vi "PID control XY vel Z R.vi"(0 "x location (um)":dbl, 1 "x polarity":bool=TRUE, 2 "y polarity":bool, 3 "z polarity":bool, 5 "y location (um)":dbl, 7 "z location (um)":dbl, 9 "measurement time":dbl, 11 "reinitialize? (F)":bool, 12 "XY vel range (mm/s)":cluster{"output high":dbl, "output low":dbl}={"output high"=1000.0, "output low"=-1000.0} {"output low" format="%.2f"; "output high" format="%.2f"}, 13 "z position range (um)":cluster{"output high":dbl, "output low":dbl}={"output high"=100.0, "output low"=-100.0} {"output low" format="%.2f"; "output high" format="%.2f"}, 14 "XY gains":T2={"chase time (ms)"=200.0, "integral time (Ti, sec)"=1.0, "derivative time (Td, sec)"=0.0} {"derivative time (Td, sec)" format="%.3f"; "integral time (Ti, sec)" format="%.3f"; "chase time (ms)" format="%.3f"}, 15 "Z gains":T1={"proportional gain (Kc)"=0.7, "integral time (Ti, sec)"=1.0, "derivative time (Td, sec)"=0.0} {"derivative time (Td, sec)" format="%.3f"; "integral time (Ti, sec)" format="%.3f"; "proportional gain (Kc)" format="%.3f"}) -> (4 "x move (um)":dbl, 6 "y move (um)":dbl, 8 "z move (um)":dbl)   [LabVIEW 2010]
uses:
  <vilib>/addons/control/pid/pid.llb/PID (DBL Array).vi
  <vilib>/addons/control/pid/NI_PID_pid.lvlib
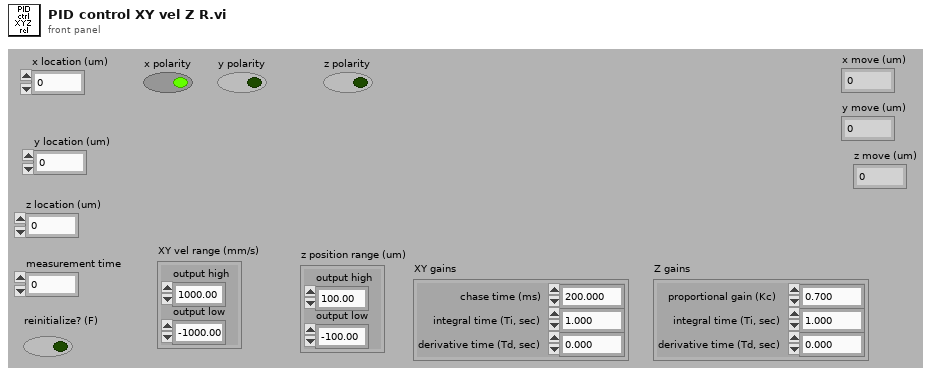
[diagram p1: front panel]
types:
  T1 = cluster{"proportional gain (Kc)":dbl, "integral time (Ti, sec)":dbl, "derivative time (Td, sec)":dbl}
  T2 = cluster{"chase time (ms)":dbl, "integral time (Ti, sec)":dbl, "derivative time (Td, sec)":dbl}
  T3 = cluster{"proportional gain (Kc)":dbl, "integral time (Ti, min)":dbl, "derivative time (Td, min)":dbl}
  T4 = cluster{"proportional gain (Kc)":dbl, "integral time (Ti, min)":dbl, "derivative time (Td, min)":dbl}[]
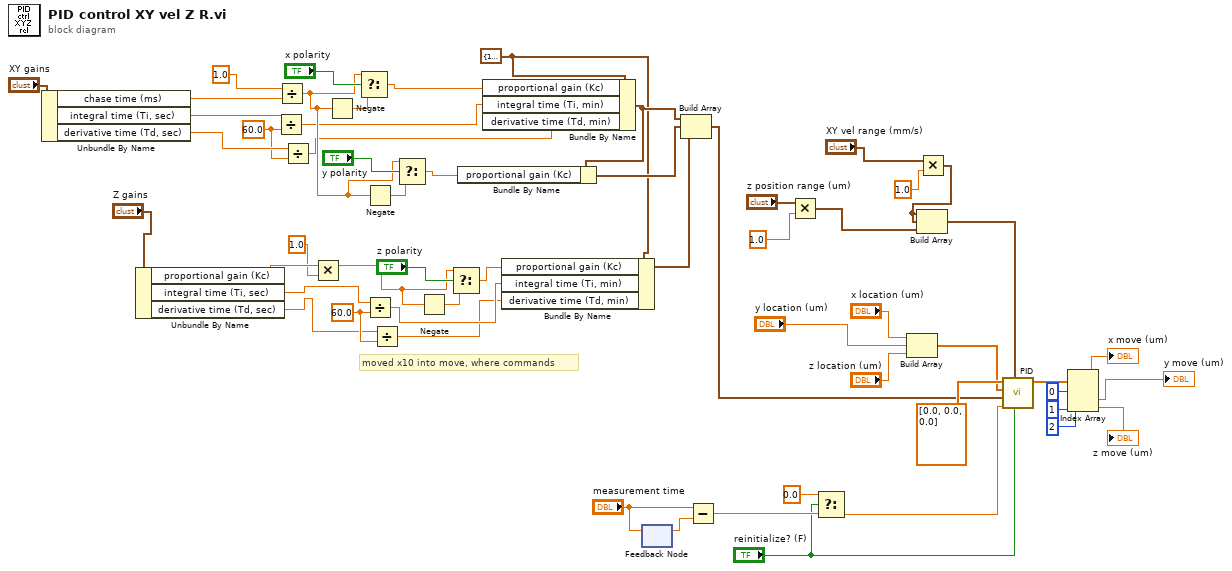
[diagram p0: block diagram]
diagram:
  w15 = 60.0 ("y")
  w50 = 60.0 ("y")
  w16 = T3 {"proportional gain (Kc)"=1.0, "integral time (Ti, min)"=0.01, "derivative time (Td, min)"=0.0} ("Z gains")
  # "moved x10 into move, where commands"
  n1 = Unbundle By Name("XY gains") -> ("chase time (ms)"=w1:dbl, "integral time (Ti, sec)"=w52:dbl, "derivative time (Td, sec)"=w51:dbl)
  n2 = Unbundle By Name("Z gains") -> ("proportional gain (Kc)"=w20:dbl, "integral time (Ti, sec)"=w14:dbl, "derivative time (Td, sec)"=w13:dbl)
  n3 = Divide(x=w52, y=w50) -> (x/y=w43:dbl)
  n4 = Divide(x=1.0, y=w1) -> (x/y=w45:dbl)
  n5 = Divide(x=w51, y=w50) -> (x/y=w42:dbl)
  n6 = Multiply(x=w20, y=1.0) -> (x*y=w18:dbl)
  n7 = Negate(x=w45) -> (-x=w48:dbl)
  n8 = Select(t=w45, s="x polarity", f=w48) -> (s? t:f=w44:dbl)
  n9 = Negate(x=w45) -> (-x=w46:dbl)
  n10 = Divide(x=w14, y=w15) -> (x/y=w12:dbl)
  n11 = Divide(x=w13, y=w15) -> (x/y=w11:dbl)
  n12 = Select(t=w45, s="y polarity", f=w46) -> (s? t:f=w41:dbl)
  n13 = Negate(x=w18) -> (-x=w21:dbl)
  n14 = Select(t=w18, s="z polarity", f=w21) -> (s? t:f=w19:dbl)
  n15 = Bundle By Name(cluster=w16, "proportional gain (Kc)"=w44, "integral time (Ti, min)"=w43, "derivative time (Td, min)"=w42) -> (w40:T3)
  n16 = Bundle By Name(cluster=w40, "proportional gain (Kc)"=w41) -> (w39:T3)
  n17 = Bundle By Name(cluster=w16, "proportional gain (Kc)"=w19, "integral time (Ti, min)"=w12, "derivative time (Td, min)"=w11) -> (w37:T3)
  n18 = feedback-in #1("measurement time") -> ()
  n19 = feedback #1() -> (w55:dbl)  [unwired: 1 in]
  n20 = Build Array(w40, w39, w37) -> (w36:T4)
  n21 = Subtract(x="measurement time", y=w55) -> (x-y=w54:dbl)
  n22 = Multiply(x="z position range (um)", y=1.0 ("measurement time")) -> (x*y=w30:cluster{"output high":dbl, "output low":dbl})
  n23 = Select(t=0.0, s="reinitialize? (F)", f=w54) -> (s? t:f=w7:dbl)
  n24 = Build Array("x location (um)", "y location (um)", "z location (um)") -> (w29:dbl[])
  n25 = Multiply(x="XY vel range (mm/s)", y=1.0 ("measurement time")) -> (x*y=w8:cluster{"output high":dbl, "output low":dbl})
  n26 = Build Array(w8, w8, w30) -> (w28:cluster{"output high":dbl, "output low":dbl}[])
  n27 = call-poly <vilib>:"PID.vi"("reinitialize? (F)"="reinitialize? (F)", "output range"=w28, "dt (s)"=w7, "PID gains"=w36, "process variable"=w29, "setpoint"=dbl[] [0.0, 0.0, 0.0]) -> ("output"=w27:dbl[])  [unwired: 4 in, 1 out]
  n28 = Index Array(array=w27, index #1=0 ("index"), index #2=1 ("index"), index #3=2 ("index")) -> (element #1=→"x move (um)":dbl, element #2=→"y move (um)":dbl, element #3=→"z move (um)":dbl)
